vi "On_tx_rx_flexray_event.vi"(4 "Variant":variant, 5 "Event Data":cluster{"AObj":refnum<k24>, "AData":refnum<k24>}, 6 "Control Ref":refnum<k24>, 7 "Event Common Data":T1) -> (1 "Event Data Out":cluster{"AData":refnum<k24>})   [LabVIEW 2018]
uses:
  <vilib>/Utility/error.llb/whitespace.ctl
  D:/LabVIEW/TSMaster_FlexRay_Labview/Interop.TSMasterAPI.dll
  Interop.TSMasterAPI.dll
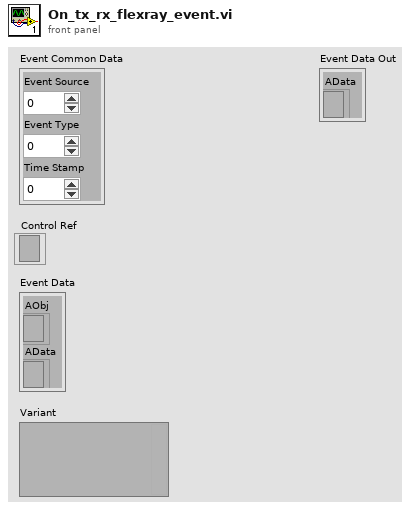
[diagram p1: front panel]
types:
  T1 = cluster{"Event Source":i32, "Event Type":u32, "Time Stamp":u32}
  T2 = typedef "whitespace.ctl" = u16
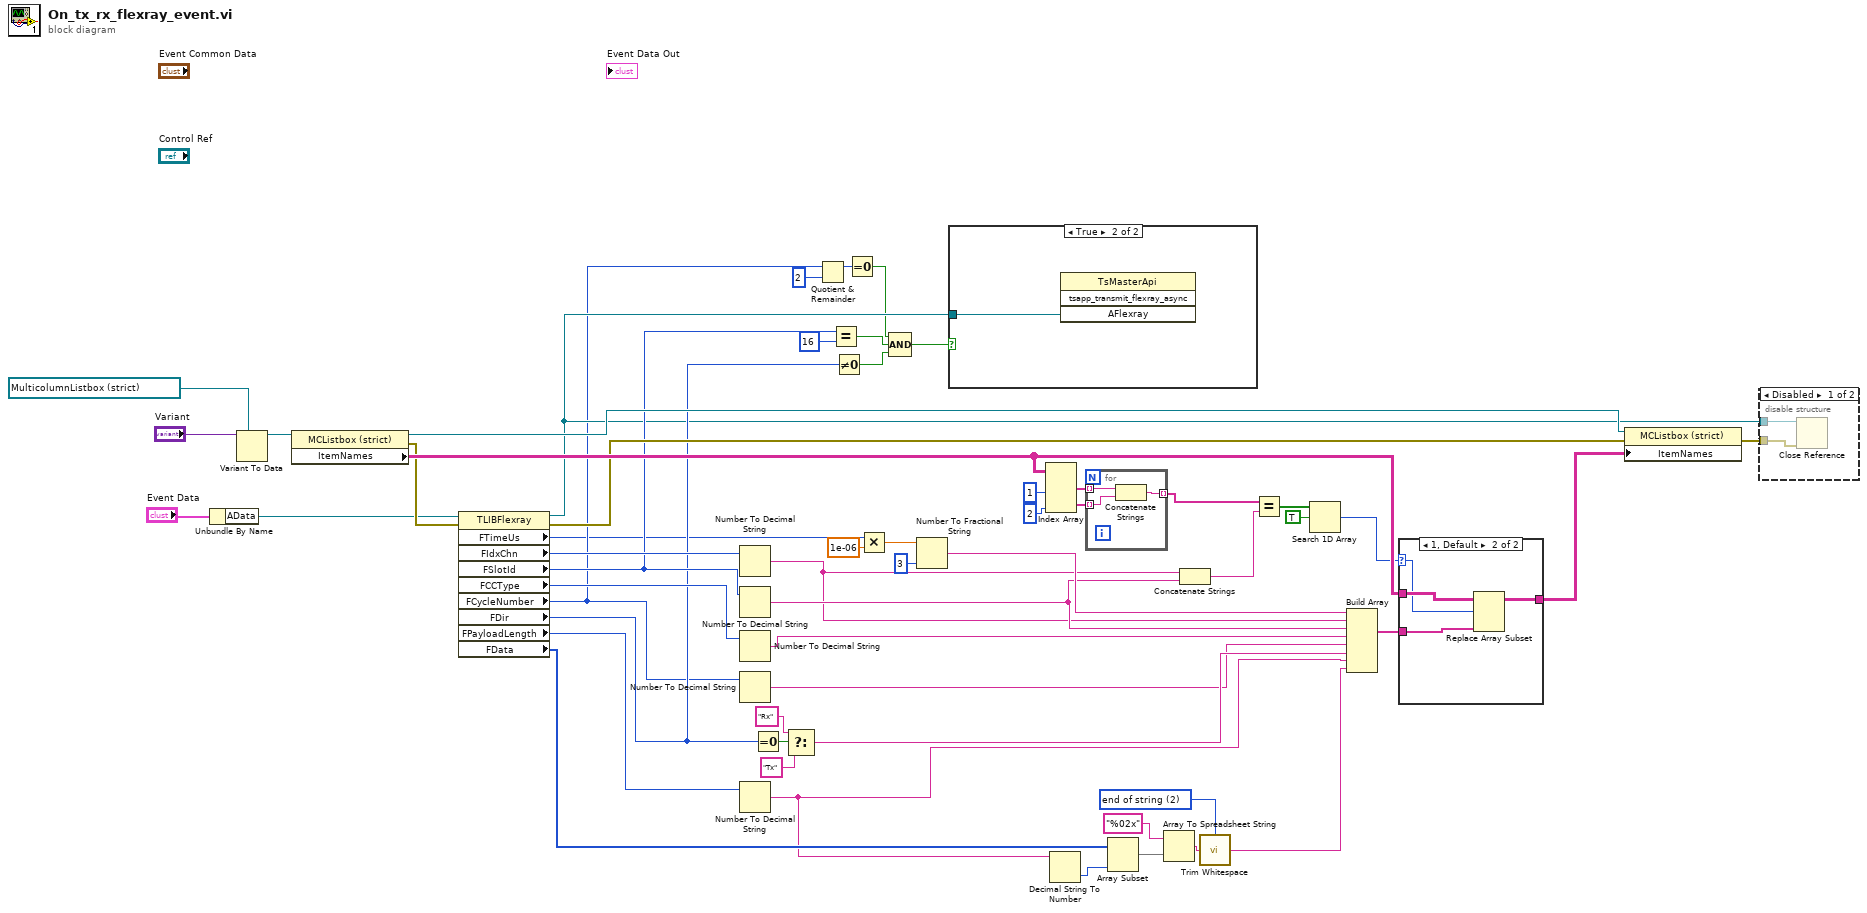
[diagram p0: block diagram]
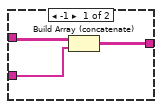
[diagram p4: hidden frame]
diagram:
  w48 = T2 2 items=["both", "start of string", "end of string"] ("location (both)")
  n1 = Unbundle By Name("Event Data") -> ("AData"=w13:refnum<k24>)
  n2 = Variant To Data(type=refnum<vi> refnum ("FlexRayFrame"), Variant="Variant") -> (data=w53:refnum<vi>)  [unwired: 1 in, 1 out]
  n3 = property class="MCListbox (strict)"(reference=w53) -> (reference out=w51:refnum<vi>, error out=w50:errorcluster, "ItemNames"=w52:string[][])  [unwired: 1 in]
  n4 = property class="TLIBFlexray"(reference=w13, error in=w50) -> (reference out=w6:refnum<k24>, error out=w17:errorcluster, "FTimeUs"=w1:u64, "FIdxChn"=w34:u8, "FSlotId"=w12:u16, "FCCType"=w33:u8, "FCycleNumber"=w5:u8, "FDir"=w10:u8, "FPayloadLength"=w35:u8, "FData"=w36:u8[])
  n5 = Number To Decimal String(number=w34) -> (decimal integer string=w14:string)  [unwired: 1 in]
  n6 = Number To Decimal String(number=w12) -> (decimal integer string=w22:string)  [unwired: 1 in]
  n7 = Number To Decimal String(number=w33) -> (decimal integer string=w28:string)  [unwired: 1 in]
  n8 = Number To Decimal String(number=w5) -> (decimal integer string=w21:string)  [unwired: 1 in]
  n9 = Number To Decimal String(number=w35) -> (decimal integer string=w26:string)  [unwired: 1 in]
  n10 = Equal To 0?(x=w10) -> (x = 0?=w32:bool)
  n11 = Select(t="Rx", s=w32, f="Tx") -> (s? t:f=w27:string)
  n12 = Quotient & Remainder(x=w5, y=u8 2) -> (x-y*floor(x/y)=w3:u8)  [unwired: 1 out]
  n13 = Equal?(x=w12, y=u16 16) -> (x = y?=w9:bool)
  n14 = Not Equal To 0?(x=w10) -> (x != 0?=w8:bool)
  n15 = Equal To 0?(x=w3) -> (x = 0?=w2:bool)
  n16 = Multiply(x=w1, y=1e-06) -> (x*y=w39:dbl)
  n17 = Compound Arithmetic op=AND(w2, w9, w8) -> (w7:bool)
  n18 = Number To Fractional String(number=w39, precision (6)=i16 3) -> (F-format string=w43:string)  [unwired: 2 in]
  n19 = case shown="True" w7 {
    tunnel: w6 -> [_ w57]
    frame False {
    }
    frame True {
      n20 = invoke class="TsMasterApi" method="tsapp_transmit_flexray_async"("AFlexray"=w57) -> ()  [unwired: 3 in, 4 out]
    }
  }
  n21 = Index Array(array=w52, index (col) #1=1 ("disabled index (col)"), index (col) #2=2 ("index (col)")) -> (element #1=w25:string[], element #2=w24:string[])  [unwired: 2 in]
  n22 = Decimal String To Number(string=w26) -> (number=w44:i32)  [unwired: 2 in, 1 out]
  n23 = for {
    tunnel: w25 -> [w60] mode=indexing
    tunnel: w24 -> [w59] mode=indexing
    tunnel: [w58] -> w20 mode=indexing
    n24 = Concatenate Strings(w60, w59) -> (w58:string)
  }
  n25 = Array Subset(array=w36, length=w44) -> (w45:u8[])  [unwired: 1 in]
  n26 = Array To Spreadsheet String(array=w45, 3:"%02x" ("format string")) -> (spreadsheet string=w47:string)  [unwired: 1 in]
  n27 = Concatenate Strings(w14, w22) -> (w19:string)
  n28 = call <vilib>:"Trim Whitespace.vi"("string"=w47, "location (both)"=w48) -> ("trimmed string"=w15:string)
  n29 = Equal?(x=w20, y=w19) -> (x = y?=w18:bool[])
  n30 = Search 1D Array(1D array=w18, element=TRUE) -> (index of element=w23:i32)  [unwired: 1 in]
  n31 = Build Array(w43, w14, w22, w28, w21, w27, w26, w15) -> (w41:string[])
  n32 = case shown="1, Default" w23 {
    selector: w23 -> [_ w64]
    tunnel: w41 -> [w62 w66]
    tunnel: w52 -> [w63 w67]
    tunnel: [w61 w65] -> w49
    frame -1 {
      n33 = Build Array (concatenate)(w63, w62) -> (w61:string[][])
    }
    frame 1, Default {
      n34 = Replace Array Subset(array=w67, new element=w66, index (row)=w64) -> (w65:string[][])  [unwired: 1 in]
    }
  }
  n35 = property class="MCListbox (strict)"(reference=w51, error in=w17, "ItemNames"=w49) -> (error out=w16:errorcluster)  [unwired: 1 out]
  n36 = disable-structure shown="Disabled" {
    disable-tunnel: w6 -> [w69 _]
    disable-tunnel: w16 -> [w68 _]
    frame Disabled {
      n37 = Close Reference(reference=w69, error in (no error)=w68) -> ()  [unwired: 1 out]
    }
    frame Enabled {
    }
  }
